vi "Caraya_Git Version.vi"() -> ()   [LabVIEW 2020]
uses:
  <vilib>/AppBuilder/AB_API_Simple/Build Specification Version.ctl
  PPL/HDH.ProjectBuilder.lvlibp/Class/Set Version from Git Tag/Set Version from Git Tag.lvclass
  PPL/HDH.ProjectBuilder.lvlibp/Class/Project Builder/Project Builder.lvclass
  PPL/HDH.ProjectBuilder.lvlibp/Class/Set Version from Git Tag/Version Data/Version Data.lvclass
  <vilib>/AppBuilder/AB_API_Simple/Set Build Specification Version (path).vi
  PPL/Caraya.lvlibp/1abvi3w/vi.lib/addons/_JKI Toolkits/Caraya/classes/Assert/Assert True.vi
  PPL/Caraya.lvlibp/1abvi3w/vi.lib/addons/_JKI Toolkits/Caraya/classes/Assert/Assert Not Error.vi
  <vilib>/AppBuilder/AB_API_Simple/Get Build Specification Version (path).vi
  PPL/Caraya.lvlibp/1abvi3w/vi.lib/addons/_JKI Toolkits/Caraya/classes/Assert/Assert Equal Value_Variant.vi
  PPL/HDH.ProjectBuilder.lvlibp/Class/Project Action/Project Action.lvclass
  PPL/Caraya.lvlibp/1abvi3w/vi.lib/addons/_JKI Toolkits/Caraya/classes/Assert/Assert.lvclass
  PPL/Caraya.lvlibp/1abvi3w/vi.lib/addons/_JKI Toolkits/Caraya/classes/Test/Test.lvclass
  <vilib>/AppBuilder/AB_API_Simple/NI_App_Builder_API.lvlib
  C:/Current projects/WS/PPL/HDH.ProjectBuilder.lvlibp/Class/Project Action/Project Action.lvclass
panel:
  out "Build Specification Version":T1
  out "error out":errorcluster
  in  "error in (no error)":errorcluster
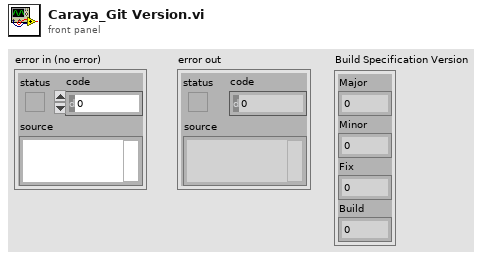
[diagram p1: front panel]
types:
  T1 = typedef "NI_App_Builder_API.lvlib/Build Specification Version.ctl" = cluster{"Major":u16, "Minor":u16, "Fix":u16, "Build":u16}
  T2 = typedef "HDH.ProjectBuilder.lvlibp/HDH.ProjectBuilder_NI_App_Builder_API.lvlib/HDH.ProjectBuilder_Build Specification Version.ctl" = cluster{"Major":u16, "Minor":u16, "Fix":u16, "Build":u16}
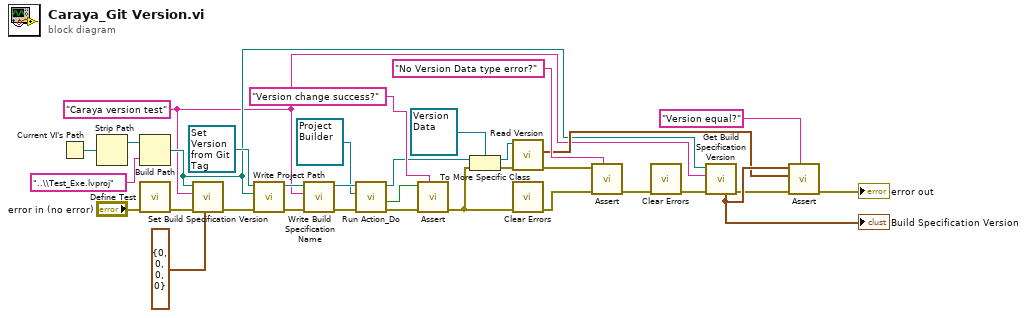
[diagram p0: block diagram]
diagram:
  w3 = "Caraya version test" ("Build Specification Name")
  n1 = Current VI's Path() -> (path=w24:path)
  n2 = Strip Path(path=w24) -> (stripped path=w23:path)  [unwired: 1 out]
  n3 = Build Path(base path=w23, name or relative path="..\\Test_Exe.lvproj") -> (appended path=w6:path)
  n4 = call "Define Test.vi"("error in (no error)"="error in (no error)") -> ("error out"=w5:errorcluster)  [unwired: 10 in]
  n5 = call-poly <vilib>:"Set Build Specification Version.vi"("Build Specification Version"=T1 {"Major"=0, "Minor"=0, "Fix"=0, "Build"=0}, "error in (no error)"=w5, "Name of build specification"=w3, "Path to project"=w6) -> ("error out"=w4:errorcluster)  [unwired: 7 in]
  n6 = call "Write Project Path.vi"("error in (no error)"=w4, "Project Path"=w6, "Project Action in"=refnum<class "Set Version from Git Tag.lvclass"> refnum ("HDH.ProjectBuilder.lvlibp:Set Version from Git Tag.lvclass")) -> ("error out"=w29:errorcluster, "Project Action out"=w32:refnum<class "Set Version from Git Tag.lvclass">)  [unwired: 7 in]
  n7 = call "Write Build Specification Name.vi"("error in (no error)"=w29, "Build Specification Name"=w3, "Set Version from Git Tag in"=w32) -> ("error out"=w28:errorcluster, "Set Version from Git Tag out"=w31:refnum<class "Set Version from Git Tag.lvclass">)  [unwired: 7 in]
  n8 = call-dynamic "Run Action_Do.vi"("error in (no error)"=w28, "Project Builder in"=refnum<class "Project Builder.lvclass"> refnum, "Set Version from Git Tag"=w31) -> ("error out"=w17:errorcluster, "Success?"=w27:bool, "Report"=w1:refnum<class "Report Data.lvclass">)  [unwired: 6 in]
  n9 = call-poly "Assert.vi"("Label"="Version change success?", "error in (no error)"=w17, "True?"=w27) -> ("error out"=w13:errorcluster)  [unwired: 8 in]
  n10 = To More Specific Class(target class=refnum<class "Version Data.lvclass"> refnum ("HDH.ProjectBuilder.lvlibp:Version Data.lvclass"), reference=w1, error in=w13) -> (specific class reference=w19:refnum<class "Version Data.lvclass">, error out=w20:errorcluster)
  n11 = call "Read Version.vi"("error in (no error)"=w20, "Version Data in"=w19) -> ("error out"=w18:errorcluster, "Build Specification Version"=w11:T2)  [unwired: 7 in, 1 out]
  n12 = call <vilib>:"Clear Errors.vi"("error in (no error)"=w13) -> ("error out"=w7:errorcluster)  [unwired: 5 in, 1 out]
  n13 = call-poly "Assert.vi"("Label"="No Version Data type error?", "error in (no error)"=w7, "Not Error?"=w18) -> ("error out"=w15:errorcluster)  [unwired: 8 in]
  n14 = call <vilib>:"Clear Errors.vi"("error in (no error)"=w15) -> ("error out"=w14:errorcluster)  [unwired: 5 in, 1 out]
  n15 = call-poly <vilib>:"Get Build Specification Version.vi"("error in (no error)"=w14, "Name of build specification"=w3, "Path to project"=w6) -> ("error out"=w9:errorcluster, "Build Specification Version"=w12:T1)  [unwired: 7 in]
  "Build Specification Version" <- w12
  n16 = call-poly "Assert.vi"("Label"="Version equal?", "error in (no error)"=w9, "Y"=w11, "X"=w12) -> ("error out"=→"error out":errorcluster)  [unwired: 7 in]
